vi "Global_CMD_Drive.vi"() -> ()   [LabVIEW 2017]
uses:
  TypeDef/CLUSTER_CMD_WC_Drive.ctl
  TypeDef/ENUM_WC_Drive_DriveMode.ctl
  TypeDef/CLUSTER_Drive_ACT Loop_VBus Data.ctl
  TypeDef/CLUSTER_X and Y.ctl
  TypeDef/CLUSTER_Drive_ACT Loop_Profile Data.ctl
panel:
  in  "CMD_Drive_Data":T1
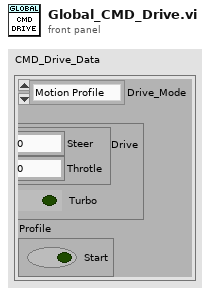
[diagram p1: front panel]
types:
  T1 = typedef "CLUSTER_CMD_WC_Drive.ctl" = cluster{"Drive_Mode":T2, "VBus":T3, "Profile":T5}
  T2 = typedef "ENUM_WC_Drive_DriveMode.ctl" = enum16{"Motion Profile", "VBus", "Stop"}
  T3 = typedef "CLUSTER_Drive_ACT Loop_VBus Data.ctl" = cluster{"Drive":T4, "Turbo":bool}
  T4 = typedef "CLUSTER_X and Y.ctl" = cluster{"Steer":dbl, "Throtle":dbl}
  T5 = typedef "CLUSTER_Drive_ACT Loop_Profile Data.ctl" = cluster{"Start":bool}
diagram:
